vi "SeCrTs-PPSU Waveform.vi"(9 "Numeric":i32, 10 "Numeric 2":i32, 11 "Numeric 3":i32) -> (3 "Array":waveform(dbl)[](array[waveform]))   [LabVIEW 2022 SP3]
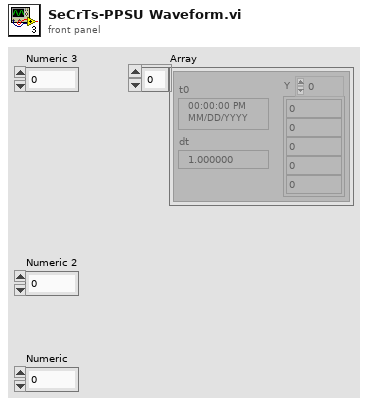
[diagram p1: front panel]
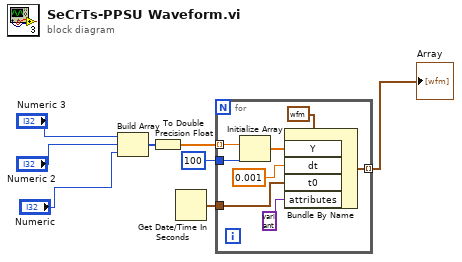
[diagram p0: block diagram]
diagram:
  n1 = Build Array("Numeric 3", "Numeric 2", "Numeric") -> (w5:i32[])
  n2 = To Double Precision Float(number=w5) -> (double precision float=w7:dbl[])
  n3 = Get Date/Time In Seconds() -> (seconds since 1Jan1904=w1:timestamp)
  n4 = for {
    tunnel: w7 -> [w16] mode=indexing
    tunnel: 100 ("dimension size") -> [w15]
    tunnel: [w11] -> w8 mode=indexing
    tunnel: w1 -> [w9]
    n5 = Initialize Array(w16, w15) -> (w14:dbl[])
    n6 = Bundle By Name(cluster=waveform(dbl) {"t0"=timestamp(0 s since 1904-01-01), "dt"=1.0, "Y"=[]} ("waveform"), "Y"=w14, "dt"=0.001, "t0"=w9, "attributes"=variant) -> (w11:waveform(dbl))
  }
  "Array" <- w8
